vi "dfd_Calculate Bound.vi"(1 "rect":T1) -> (0 "Bounds":cluster{"Width":i16, "Height":i16})   [LabVIEW 2017, in "NI_DigFilter_Process.lvlib"]
uses:
  <vilib>/addons/Digital Filter Design/NI_DigFilter_Process.lvlib
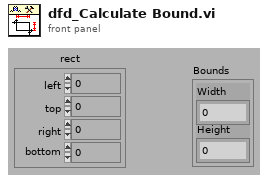
[diagram p1: front panel]
types:
  T1 = cluster{"left":i16, "top":i16, "right":i16, "bottom":i16}
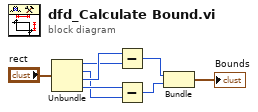
[diagram p0: block diagram]
diagram:
  n1 = Unbundle("rect") -> ("left"=w6:i16, "top"=w4:i16, "right"=w7:i16, "bottom"=w5:i16)
  n2 = Subtract(x=w7, y=w6) -> (x-y=w3:i16)
  n3 = Subtract(x=w5, y=w4) -> (x-y=w2:i16)
  n4 = Bundle(w3, w2) -> (→"Bounds":cluster{i16, i16})  [unwired: 1 out]
